vi "PageUI.vi"() -> ()   [LabVIEW 2015, in "Page.lvclass"]
uses:
  Page.lvclass
  <vilib>/NI/Configuration Framework/Node/NodeRef.ctl
  <vilib>/NI/Configuration Framework/Node/NISE_CEF_Node.lvclass
  <vilib>/NI/AMC/Message Queue.ctl
  <vilib>/NI/AMC/Message.ctl
  <vilib>/NI/Tools/Keyed Array/KeyedArray.ctl
  <vilib>/NI/Configuration Framework/Node/UserEventRef.ctl
  <vilib>/NI/Configuration Framework/Controls/EventCluster.ctl
  Page.lvclass/Page.ctl
  XML Controls/help.ctl
  XML Controls/Path Cluster.ctl
  Read General Page Properties.vi
  Write General Page Properties.vi
  <vilib>/NI/AMC/Create Single Message.vi
  <vilib>/NI/AMC/Update Message Routing Info.vi
  <vilib>/NI/AMC/Send Message.vi
  <vilib>/NI/AMC/AMC.lvlib
  Configuration Tool.lvlib
  <vilib>/NI/Tools/Keyed Array/Tools_KeyedArray.lvlib
  <vilib>/NI/Configuration Framework/NISE_CEF_TreeControl.lvlib
panel:
  in  "Help Section":string
  in  "Help File Type":enum16{"chm", "other"}(ring)
  in  "Host Path to Help File":path
  in  "Paste Action":T1(ring)
  in  "Copy Action":enum16{"copy", "disabled"}(ring)
  in  "Host Path to Page VI":path
  in  "Host Path to Broken Glyph":path
  in  "Host Path to Inactive Glyph":path
  in  "Host Path to Glyph":path
  in  "Multiselect":bool
  in  "Alphabetical":bool
  in  "Delete":bool
  in  "Rename":bool
  in  "GUID":string="9b525fa0-4d4a-4ec1-902b-bfeef88ebbcc"
  in  "Page Name":string
  in  "user event":T2
  in  "main queue":T3
  in  "node ref":T4
  # "General Settings"
  # "Advanced Settings"
  # "Help File Settings"
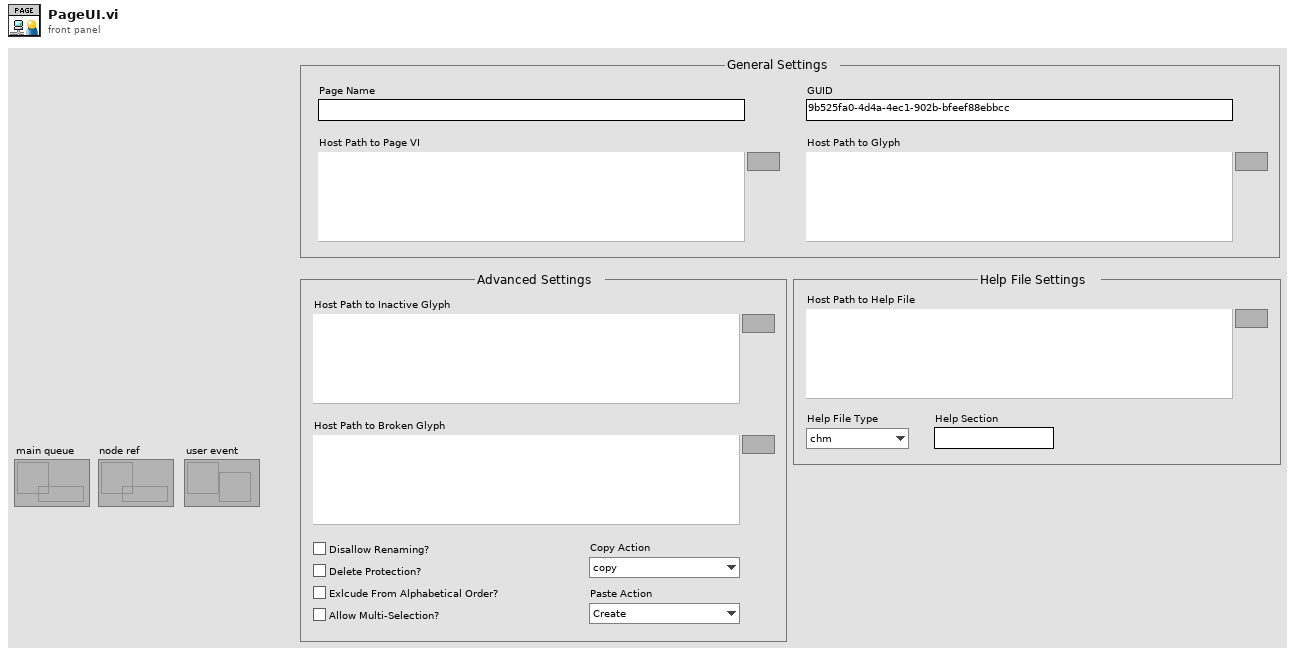
[diagram p1: front panel]
types:
  T1 = enum16{"Create", "CreatIfNotExists_GUID", "CreatIfNotExists_Name", "Replace", "Dialog"}
  T2 = typedef "NISE_CEF_Node.lvclass/UserEventRef.ctl" = refnum<user-event>
  T3 = typedef "AMC.lvlib/Message Queue.ctl" = refnum<queue>
  T4 = typedef "NISE_CEF_Node.lvclass/NodeRef.ctl" = refnum<data-value>
  T5 = typedef "Page Properties.ctl" = cluster{"Name":string, "Disallow Renaming":bool, "Delete Protection":bool, "Exlcude from Alphabetical order":bool, "Allow Multi-Selection":bool, "GUID":string, "Parent GUIDs":string[], "Glyph":T6, "Inactive Glyph":T6, "Broken Glyph":T6, "Item to Launch":T6, "Additional Information":string, "Copy":enum16{"copy", "disabled"}, "Paste":enum16{"Create", "CreatIfNotExists_GUID", "CreatIfNotExists_Name", "Replace", "Dialog"}, "Help":T7}
  T6 = typedef "Path Cluster.ctl" = cluster{"Path":path, "Path Type":enum16{"Absolute", "To Base", "To Common Doc Dir", "To Application Data Dir"}}
  T7 = typedef "help.ctl" = cluster{"Item to Launch":T6, "Section":string, "File Type":enum16{"chm", "other"}}
  T8 = enum16{"Absolute", "To Base", "To Common Doc Dir", "To Application Data Dir"}
  T9 = typedef "Configuration Tool.lvlib/help.ctl" = cluster{"Item to Launch":T10, "Section":string, "File Type":enum16{"chm", "other"}}
  T10 = typedef "Configuration Tool.lvlib/Path Cluster.ctl" = cluster{"Path":path, "Path Type":enum16{"Absolute", "To Base", "To Common Doc Dir", "To Application Data Dir"}}
  T11 = cluster{path, "VS Enum Out":enum16{"Absolute", "To Base", "To Common Doc Dir", "To Application Data Dir"}}
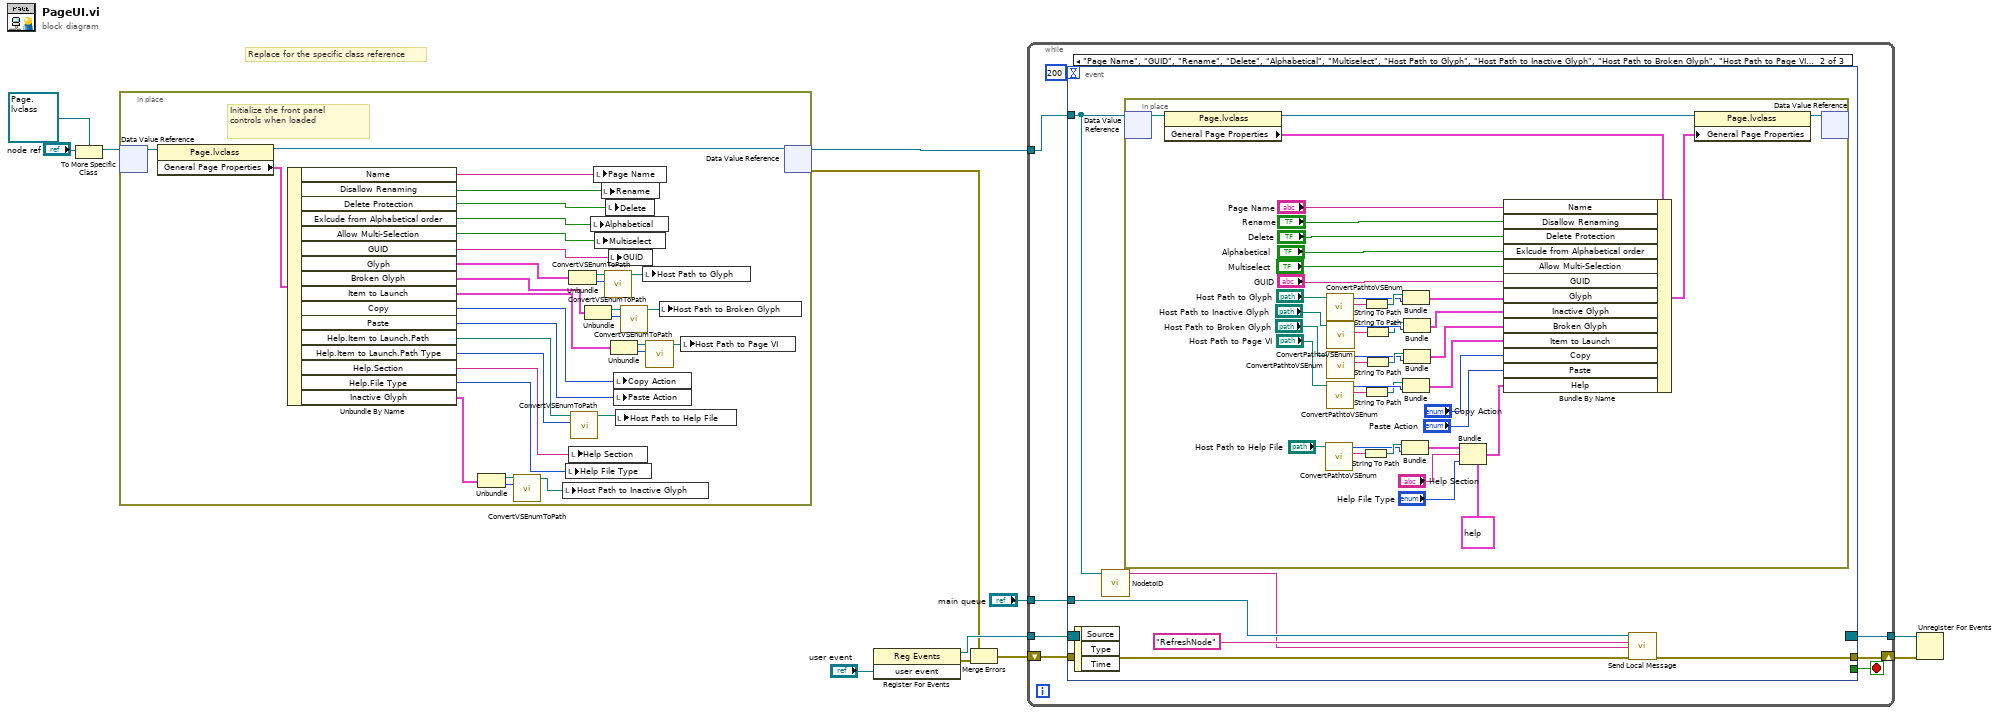
[diagram p0: block diagram]
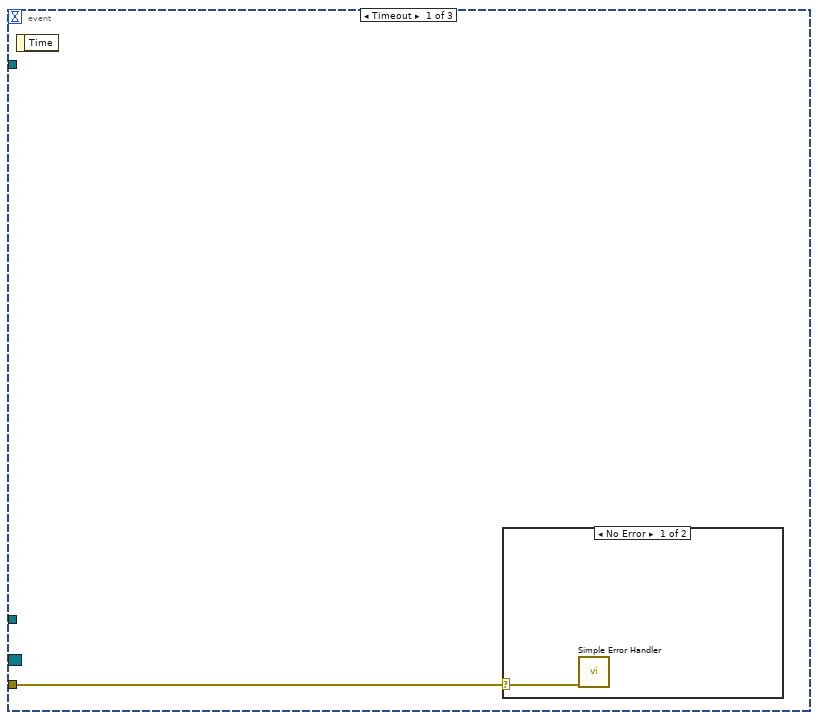
[diagram p2: hidden frame]
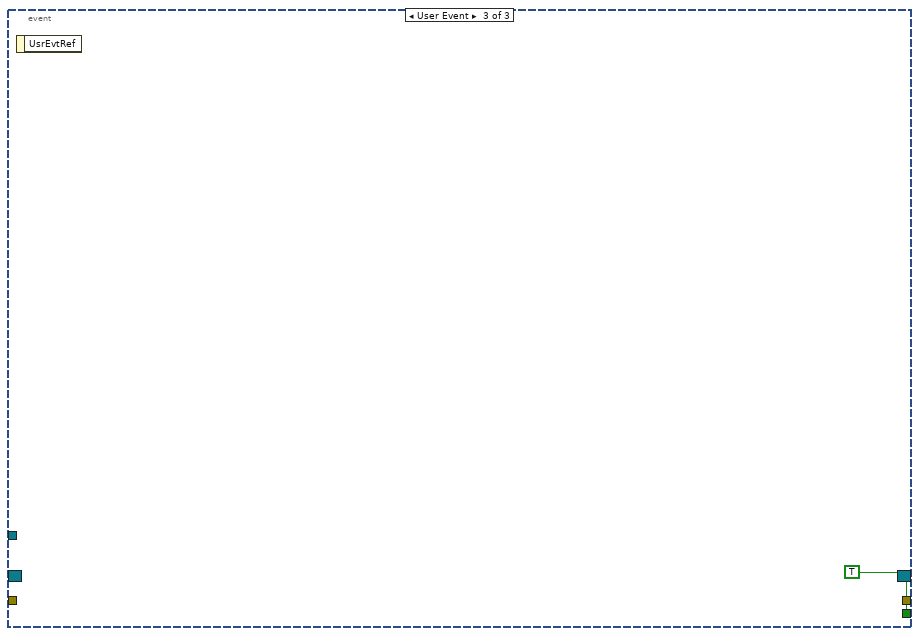
[diagram p4: hidden frame]
diagram:
  # "Replace for the specific class reference"
  n1 = To More Specific Class(target class=refnum<data-value> refnum ("data value reference"), reference="node ref") -> (specific class reference=w5:refnum<data-value>)  [unwired: 1 in, 1 out]
  n2 = in-place {
    # "Initialize the front panel controls when loaded"
    n3 = in-place-dvr #1(w5) -> (w44:refnum<class "Page.lvclass">)  [unwired: 1 out]
    n4 = property class="Page.lvclass"(reference=w44) -> (reference out=w43:refnum<class "Page.lvclass">, "General Page Properties"=w42:T5)  [unwired: 1 in, 1 out]
    n5 = Unbundle By Name(w42) -> ("Name"=w41:string, "Disallow Renaming"=w40:bool, "Delete Protection"=w39:bool, "Exlcude from Alphabetical order"=w38:bool, "Allow Multi-Selection"=w37:bool, "GUID"=w36:string, "Glyph"=w17:T6, "Broken Glyph"=w31:T6, "Item to Launch"=w28:T6, "Copy"=w24:enum16{"copy", "disabled"}, "Paste"=w23:T1, "Help.Item to Launch.Path"=w22:path, "Help.Item to Launch.Path Type"=w21:T8, "Help.Section"=w19:string, "Help.File Type"=w18:enum16{"chm", "other"}, "Inactive Glyph"=w15:T6)
    n6 = Unbundle(w15) -> ("Path"=w14:path, "Path Type"=w13:T8)
    n7 = call "ConvertVSEnumToPath.vi"("Source.Path Type"=w13, "Path In"=w14) -> ("appended path"=w16:path)  [unwired: 9 in]
    n8 = local write "Host Path to Inactive Glyph"(w16) -> ()
    n9 = local write "Help File Type"(w18) -> ()
    n10 = Unbundle(w17) -> ("Path"=w35:path, "Path Type"=w34:T8)
    n11 = local write "Help Section"(w19) -> ()
    n12 = call "ConvertVSEnumToPath.vi"("Source.Path Type"=w21, "Path In"=w22) -> ("appended path"=w20:path)  [unwired: 9 in]
    n13 = Unbundle(w31) -> ("Path"=w25:path, "Path Type"=w32:T8)
    n14 = local write "Alphabetical"(w38) -> ()
    n15 = local write "Page Name"(w41) -> ()
    n16 = local write "Multiselect"(w37) -> ()
    n17 = local write "Rename"(w40) -> ()
    n18 = call "ConvertVSEnumToPath.vi"("Source.Path Type"=w34, "Path In"=w35) -> ("appended path"=w33:path)  [unwired: 9 in]
    n19 = local write "Delete"(w39) -> ()
    n20 = local write "GUID"(w36) -> ()
    n21 = Unbundle(w28) -> ("Path"=w27:path, "Path Type"=w29:T8)
    n22 = local write "Copy Action"(w24) -> ()
    n23 = local write "Paste Action"(w23) -> ()
    n24 = local write "Host Path to Help File"(w20) -> ()
    n25 = call "ConvertVSEnumToPath.vi"("Source.Path Type"=w32, "Path In"=w25) -> ("appended path"=w30:path)  [unwired: 9 in]
    n26 = local write "Host Path to Glyph"(w33) -> ()
    n27 = call "ConvertVSEnumToPath.vi"("Source.Path Type"=w29, "Path In"=w27) -> ("appended path"=w26:path)  [unwired: 9 in]
    n28 = local write "Host Path to Broken Glyph"(w30) -> ()
    n29 = local write "Host Path to Page VI"(w26) -> ()
    n30 = in-place-dvr #1(w43) -> (w12:refnum<data-value>, w2:errorcluster)
  }
  n31 = register-events("user event") -> (reference out=w9:refnum<event-registration>, error out=w3:errorcluster)  [unwired: 2 in]
  n32 = Merge Errors(w2, w3) -> (w1:errorcluster)
  n33 = while {
    tunnel: w12 -> [w52]
    tunnel: "main queue" -> [w51]
    tunnel: w9 -> [w49]
    tunnel: [w48] -> w8
    shift-right: [w46] -> w7
    shift-left: w1 -> [w45]
    stop <- w47 stop-if-true
    n34 = event shown="[1] \"Page Name\", \"GUID\", \"Rename\", \"Delete\", \"Alphabetical\", \"Multiselect\", \"Host Path to Glyph\", \"Host Path to Inactive Glyph\", \"Host Path to Broken Glyph\", \"Host Path to Page VI\", \"Copy Action\", \"Paste Action\", \"Host Path to Help File\", \"Help File Type\", \"Help Section\": Value Change" {
      selector: w49 -> [_ _ _]
      dyn-events: [_ _ _] -> w48
      timeout: 200 -> [_ _ _]
      tunnel: w52 -> [_ w58 _]
      tunnel: w51 -> [_ w59 _]
      tunnel: [_ _ TRUE] -> w47
      tunnel: [_ w56 _] -> w46
      tunnel: w45 -> [w53 w55 _]
      event Timeout {
        n35 = event-data() -> ()  [unwired: 1 in, 1 out]
        n36 = case shown="No Error" w53 {
          selector: w53 -> [w54 _]
          frame No Error {
            n37 = call <vilib>:"Simple Error Handler.vi"("error in (no error)"=w54) -> ()  [unwired: 4 in, 5 out]
          }
          frame Error {
          }
        }
      }
      event "Page Name", "GUID", "Rename", "Delete", "Alphabetical", "Multiselect", "Host Path to Glyph", "Host Path to Inactive Glyph", "Host Path to Broken Glyph", "Host Path to Page VI", "Copy Action", "Paste Action", "Host Path to Help File", "Help File Type", "Help Section": Value Change {
        n38 = event-data() -> ()  [unwired: 1 in, 3 out]
        n39 = call <vilib>:"NodetoID.vi"("node ref"=w58) -> ("ID"=w57:string)  [unwired: 9 in, 1 out]
        n40 = in-place {
          n41 = in-place-dvr #2(w58) -> (w101:refnum<class "Page.lvclass">)  [unwired: 1 out]
          n42 = property class="Page.lvclass"(reference=w101) -> (reference out=w100:refnum<class "Page.lvclass">, "General Page Properties"=w99:T5)  [unwired: 1 in, 1 out]
          n43 = call "ConvertPathtoVSEnum.vi"("Path In"="Host Path to Help File") -> ("Remaining Path"=w70:string, "VS Enum Out"=w68:T8)  [unwired: 9 in]
          n44 = call "ConvertPathtoVSEnum.vi"("Path In"="Host Path to Glyph") -> ("Remaining Path"=w90:string, "VS Enum Out"=w88:T8)  [unwired: 9 in]
          n45 = call "ConvertPathtoVSEnum.vi"("Path In"="Host Path to Page VI") -> ("Remaining Path"=w79:string, "VS Enum Out"=w81:T8)  [unwired: 9 in]
          n46 = call "ConvertPathtoVSEnum.vi"("Path In"="Host Path to Inactive Glyph") -> ("Remaining Path"=w85:string, "VS Enum Out"=w87:T8)  [unwired: 9 in]
          n47 = call "ConvertPathtoVSEnum.vi"("Path In"="Host Path to Broken Glyph") -> ("Remaining Path"=w84:string, "VS Enum Out"=w82:T8)  [unwired: 9 in]
          n48 = String To Path(string=w70) -> (path=w69:path)
          n49 = String To Path(string=w90) -> (path=w89:path)
          n50 = String To Path(string=w79) -> (path=w80:path)
          n51 = String To Path(string=w85) -> (path=w86:path)
          n52 = String To Path(string=w84) -> (path=w83:path)
          n53 = Bundle(w69, "VS Enum Out"=w68) -> (w66:T11)  [unwired: 1 in]
          n54 = Bundle(w89, "VS Enum Out"=w88) -> (w91:T11)  [unwired: 1 in]
          n55 = Bundle(w80, "VS Enum Out"=w81) -> (w73:T11)  [unwired: 1 in]
          n56 = Bundle(w86, "VS Enum Out"=w87) -> (w77:T11)  [unwired: 1 in]
          n57 = Bundle(w83, "VS Enum Out"=w82) -> (w75:T11)  [unwired: 1 in]
          n58 = Bundle(cluster=T9 {"Item to Launch"={"Path"=path "", "Path Type"=enum."Absolute"}, "Section"="", "File Type"=enum."chm"} ("Help"), "Item to Launch"=w66, "Section"="Help Section", "File Type"="Help File Type") -> (w62:T9)
          n59 = Bundle By Name(cluster=w99, "Name"="Page Name", "Disallow Renaming"="Rename", "Delete Protection"="Delete", "Exlcude from Alphabetical order"="Alphabetical", "Allow Multi-Selection"="Multiselect", "GUID"="GUID", "Glyph"=w91, "Inactive Glyph"=w77, "Broken Glyph"=w75, "Item to Launch"=w73, "Copy"="Copy Action", "Paste"="Paste Action", "Help"=w62) -> (w61:T5)
          n60 = property class="Page.lvclass"(reference=w100, "General Page Properties"=w61) -> (reference out=w102:refnum<class "Page.lvclass">)  [unwired: 1 in, 1 out]
          n61 = in-place-dvr #2(w102) -> ()  [unwired: 2 out]
        }
        n62 = call <vilib>:"Send Local Message.vi"("message queue in"=w59, "message name"="RefreshNode" ("Message Name"), "message value"=w57, "error in"=w55) -> ("error out"=w56:errorcluster)  [unwired: 9 in, 2 out]
      }
      event User Event {
        n63 = event-data() -> ()  [unwired: 1 in, 1 out]
      }
    }
  }
  n64 = Unregister For Events(event registration refnum=w8, error in=w7) -> ()  [unwired: 1 out]
